vi "Build Mulit Data String.vi"(8 "error in (no error)":errorcluster, 10 "2D Array":string[][](array[string]), 11 "SQLite_API in":refnum<class "SQLite_API.lvclass">) -> (0 "error out":errorcluster, 2 "Data String":string, 3 "SQLite_API out":refnum<class "SQLite_API.lvclass">)   [LabVIEW 2021, in "SQLite_API.lvclass"]
uses:
  <userlib>/John_Lib/DataBase/SQLite_API/SQLite_API.lvclass
  <userlib>/John_Lib/DataBase/SQLite_API/SQLite_API.lvclass/SQLite_API.ctl
  <userlib>/John_Lib/DataBase/DataBase_SQL/DataBase_SQL.lvclass
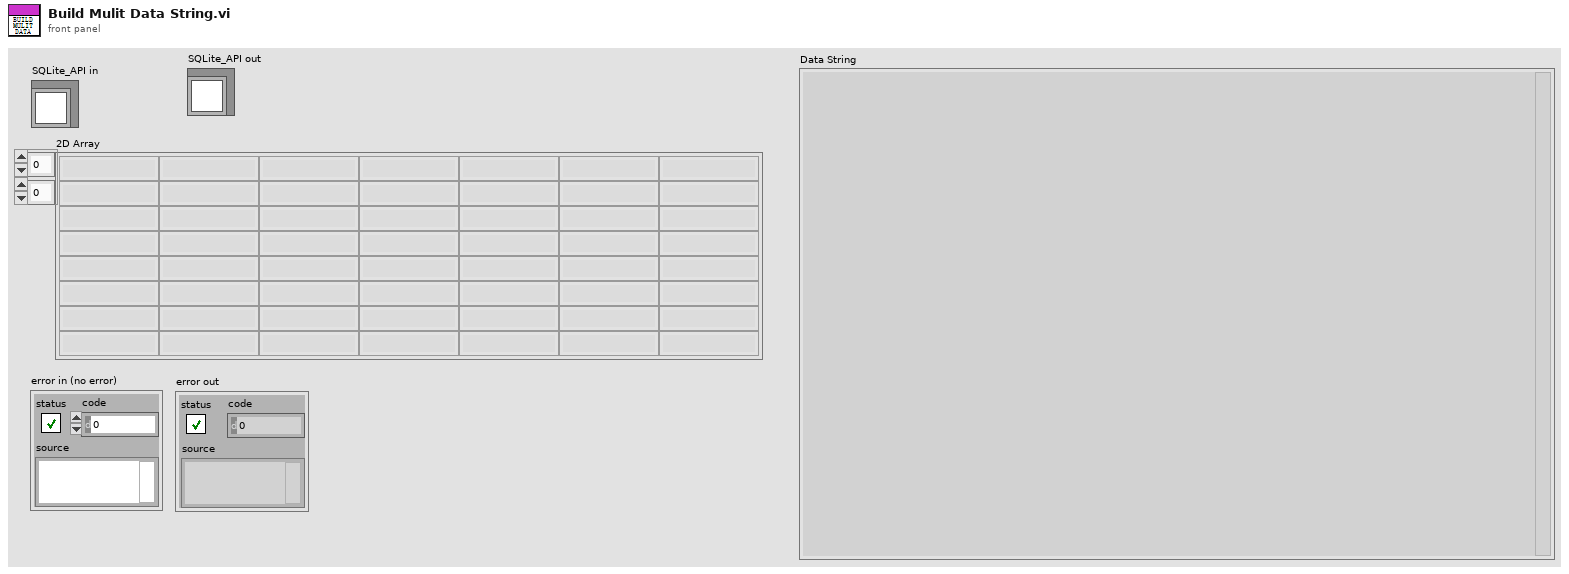
[diagram p1: front panel]
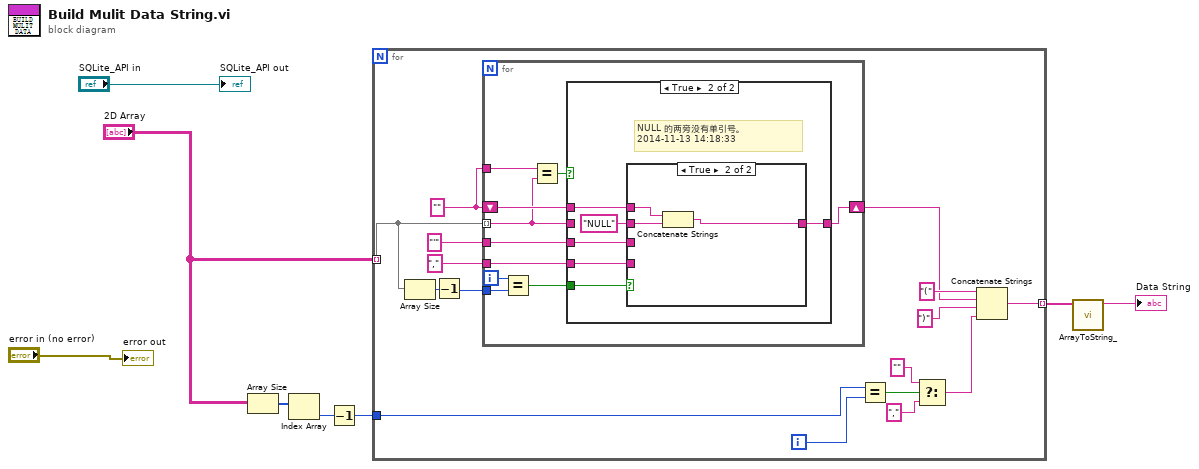
[diagram p0: block diagram]
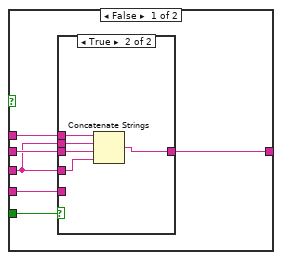
[diagram p2: hidden frame]
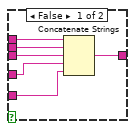
[diagram p3: hidden frame]
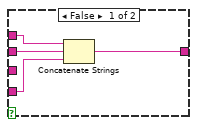
[diagram p4: hidden frame]
diagram:
  n1 = Array Size(array="2D Array") -> (size(s)=w5:i32[])
  n2 = Index Array(array=w5) -> (element=w6:i32)  [unwired: 1 in]
  n3 = Decrement(x=w6) -> (x-1=w7:i32)
  n4 = for {
    tunnel: "2D Array" -> [w10] mode=indexing
    tunnel: [w22] -> w3 mode=indexing
    tunnel: w7 -> [w21]
    i -> [w20]
    w13 = "" ("string")
    n5 = Array Size(array=w10) -> (size(s)=w15:i32)
    n6 = Decrement(x=w15) -> (x-1=w14:i32)
    n7 = for {
      tunnel: w10 -> [w27] mode=indexing
      shift-right: [w28] -> w9
      shift-left: w13 -> [w29]
      tunnel: "'" ("string") -> [w34]
      tunnel: "," ("string") -> [w33]
      tunnel: w14 -> [w31]
      tunnel: w13 -> [w26]
      i -> [w32]
      n8 = Equal?(x=w32, y=w31) -> (x = y?=w30:bool)
      n9 = Equal?(x=w26, y=w27) -> (x = y?=w25:bool)
      n10 = case shown="True" w25 {
        tunnel: w27 -> [w36 _]
        tunnel: w34 -> [w35 w57]
        tunnel: w33 -> [w40 w56]
        tunnel: w30 -> [w39 w55]
        tunnel: w29 -> [w38 w54]
        tunnel: [w37 w53] -> w28
        frame False {
          n11 = case shown="True" w39 {
            tunnel: w36 -> [w46 w51]
            tunnel: [w45 w50] -> w37
            tunnel: w35 -> [w44 w49]
            tunnel: w40 -> [w43 _]
            tunnel: w38 -> [w42 w48]
            tunnel: w35 -> [w41 w47]
            frame False {
              n12 = Concatenate Strings(w42, w41, w46, w44, w43) -> (w45:string)
            }
            frame True {
              n13 = Concatenate Strings(w48, w47, w51, w49) -> (w50:string)
            }
          }
        }
        frame True {
          # "NULL 的两旁没有单引号。\n2014-11-13 14:18:33"
          n14 = case shown="True" w55 {
            tunnel: "NULL" ("Double all the singe quotation Mark in the string") -> [w61 w64]
            tunnel: [w60 w63] -> w53
            tunnel: w57 -> [_ _]
            tunnel: w56 -> [w59 _]
            tunnel: w54 -> [w58 w62]
            frame False {
              n15 = Concatenate Strings(w58, w61, w59) -> (w60:string)
            }
            frame True {
              n16 = Concatenate Strings(w62, w64) -> (w63:string)
            }
          }
        }
      }
    }
    n17 = Equal?(x=w21, y=w20) -> (x = y?=w19:bool)
    n18 = Select(t="", s=w19, f="," ("string")) -> (s? t:f=w17:string)
    n19 = Concatenate Strings("(" ("string"), w9, ")" ("string"), w17) -> (w22:string)
  }
  n20 = call <userlib>:"ArrayToString_.vi"("Array"=w3) -> ("String"=→"Data String":string)  [unwired: 10 in]
  "error out" <- "error in (no error)"
  "SQLite_API out" <- "SQLite_API in"
